vi "NISE.Write Session.TCPIP.ConnectTimeout.vi"(8 "error in (no error)":errorcluster, 10 "Session.TCPIP.ConnectTimeout":dbl, 11 "SLSC Interface in":refnum<class "SLSC Interface.lvclass">) -> (0 "error out":errorcluster, 3 "SLSC Interface out":refnum<class "SLSC Interface.lvclass">)   [LabVIEW 2016, in "SLSC Interface.lvclass"]
uses:
  SLSC Interface.lvclass
  SLSC Interface.lvclass/SLSC Interface.ctl
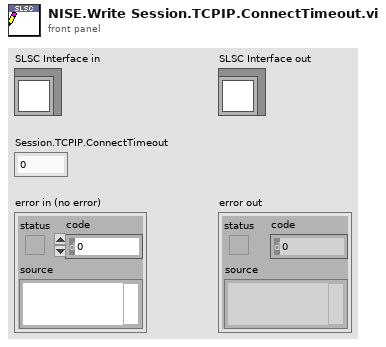
[diagram p1: front panel]
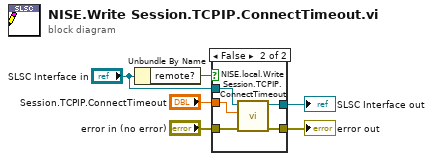
[diagram p0: block diagram]
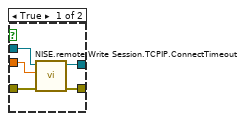
[diagram p2: hidden frame]
diagram:
  n1 = Unbundle By Name("SLSC Interface in") -> ("remote?"=w6:bool)
  n2 = case shown="False" w6 {
    tunnel: [w11 w16] -> w5
    tunnel: [w10 w15] -> w4
    tunnel: "error in (no error)" -> [w9 w14]
    tunnel: "Session.TCPIP.ConnectTimeout" -> [w8 w13]
    tunnel: "SLSC Interface in" -> [w7 w12]
    frame True {
      n3 = call "NISE.remote.Write Session.TCPIP.ConnectTimeout.vi"("error in (no error)"=w9, "Session.TCPIP.ConnectTimeout"=w8, "SLSC Remote in"=w7) -> ("error out"=w11:errorcluster, "SLSC Remote out"=w10:refnum<class "SLSC Interface.lvclass">)  [unwired: 7 in]
    }
    frame False {
      n4 = call "NISE.local.Write Session.TCPIP.ConnectTimeout.vi"("error in (no error)"=w14, "Session.TCPIP.ConnectTimeout"=w13, "SLSC Local in"=w12) -> ("error out"=w16:errorcluster, "SLSC Local out"=w15:refnum<class "SLSC Interface.lvclass">)  [unwired: 7 in]
    }
  }
  "error out" <- w5
  "SLSC Interface out" <- w4
